vi "LabVIEW_commandline.vi"() -> ()   [LabVIEW 2016]
panel:
  out "concatenated string":string
  in  "Computer Selector":u16(ring)=1 items=["AERO-06", "AERO-03"]
  in  "PD Filepath":path=path "D:/PDE Project/PDE Data/Default Data/PD.tdms"
  in  "TC Filepath":path=path "D:/PDE Project/PDE Data/Default Data/TC.tdms"
  in  "PT Filepath":path=path "D:/PDE Project/PDE Data/Default Data/PT.tdms"
  in  "Diluent":string="N2"
  in  "Menu Ring":u16(ring) items=["Manual Find", "Use Path"]
  in  "Working Directory":path=path "C:/Users/DAQ/Desktop/Mass-Flow-Calculator"
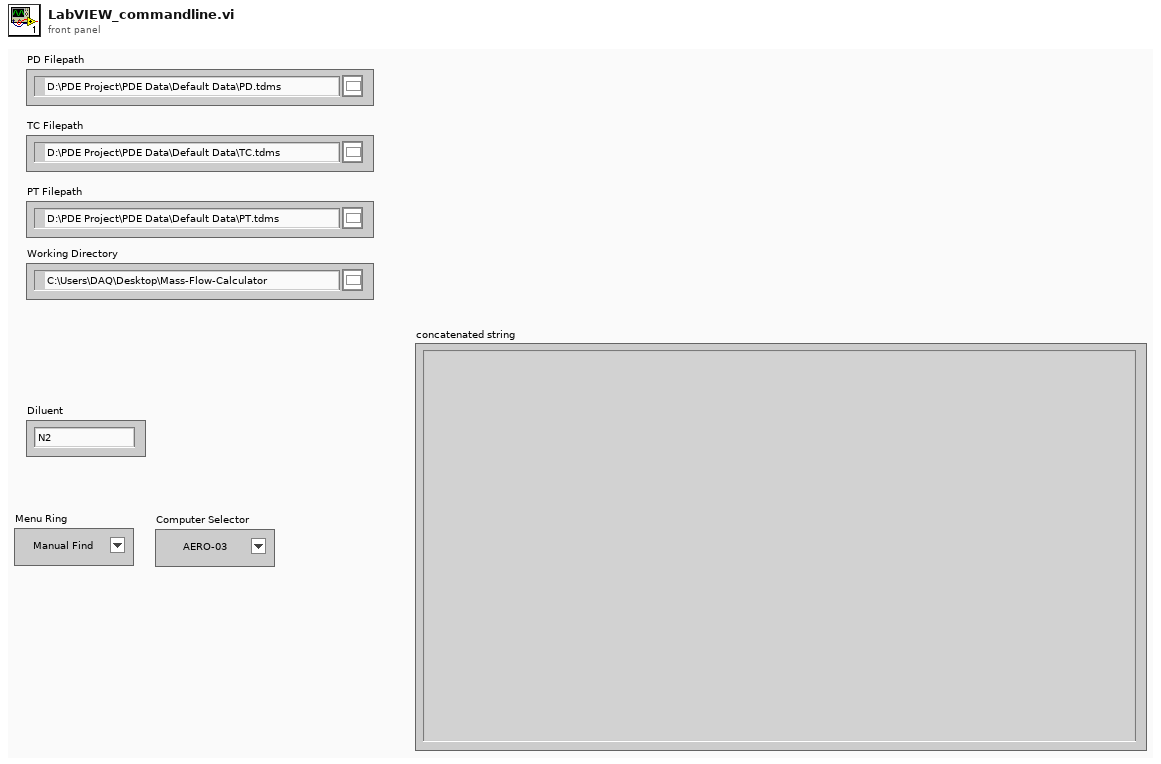
[diagram p1: front panel]
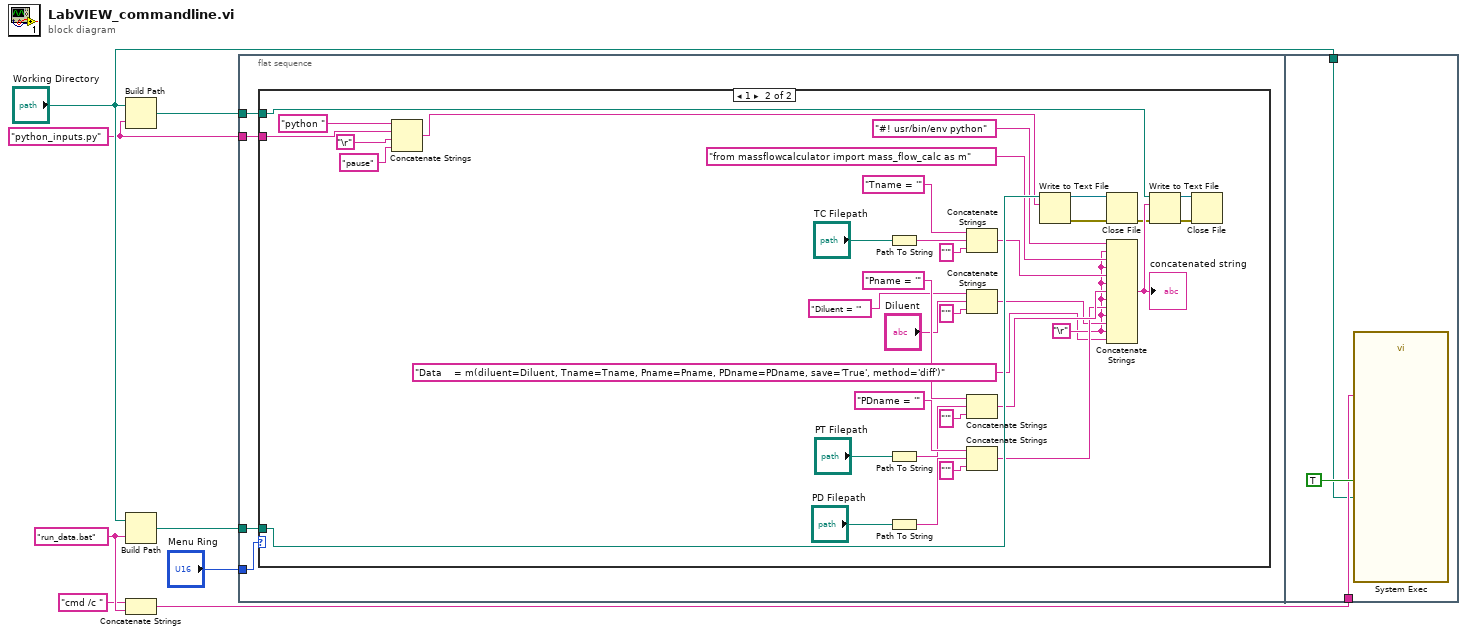
[diagram p0: block diagram]
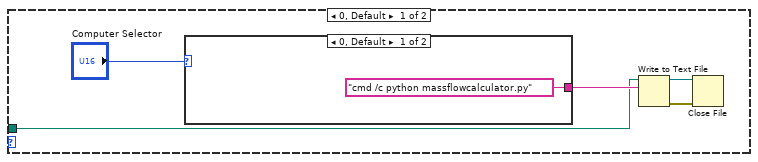
[diagram p2: hidden frame]
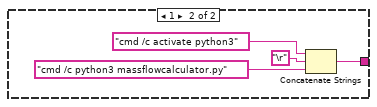
[diagram p3: hidden frame]
diagram:
  w1 = "python_inputs.py" ("name or relative path")
  w5 = "run_data.bat"
  n1 = Build Path(base path="Working Directory", name or relative path=w1) -> (appended path=w2:path)
  n2 = Build Path(base path="Working Directory", name or relative path=w5) -> (appended path=w7:path)
  n3 = Concatenate Strings("cmd /c " ("string"), w5) -> (w6:string)
  n4 = flat-sequence {
    tunnel: "Menu Ring" -> [w12]
    tunnel: w7 -> [w11]
    tunnel: w2 -> [w10]
    tunnel: w1 -> [w9]
    tunnel: w6 -> [w60]
    tunnel: "Working Directory" -> [w59]
    frame #0 {
      n5 = case shown="1" w12 {
        tunnel: w11 -> [w14 w53]
        tunnel: w10 -> [_ w28]
        tunnel: w9 -> [_ w26]
        frame 0, Default {
          n6 = case shown="0, Default" "Computer Selector" {
            tunnel: ["cmd /c python massflowcalculator.py" w19] -> w15
            frame 0, Default {
            }
            frame 1 {
              n7 = Concatenate Strings("cmd /c activate python3" ("text"), "\r", "cmd /c python3 massflowcalculator.py") -> (w19:string)
            }
          }
          n8 = Write to Text File(file (use dialog)=w14, text=w15) -> (refnum out=w16:refnum<file>, error out=w17:errorcluster)  [unwired: 2 in, 1 out]
          n9 = Close File(refnum=w16, error in=w17) -> ()  [unwired: 2 out]
        }
        frame 1 {
          w32 = "\r"
          n10 = Concatenate Strings("python " ("text"), w26, "\r", "pause" ("string")) -> (w25:string)
          n11 = Path To String(path="TC Filepath") -> (string=w46:string)
          n12 = Path To String(path="PT Filepath") -> (string=w41:string)
          n13 = Path To String(path="PD Filepath") -> (string=w40:string)
          n14 = Concatenate Strings("Tname = '" ("string"), w46, "'" ("string")) -> (w39:string)
          n15 = Concatenate Strings("Diluent = '" ("string"), "Diluent", "'" ("string")) -> (w33:string)
          n16 = Concatenate Strings("Pname = '" ("string"), w41, "'" ("string")) -> (w38:string)
          n17 = Concatenate Strings("PDname = '" ("string"), w40, "'" ("string")) -> (w37:string)
          n18 = Write to Text File(file (use dialog)=w53, text=w25) -> (refnum out=w54:refnum<file>, error out=w55:errorcluster)  [unwired: 2 in, 1 out]
          n19 = Close File(refnum=w54, error in=w55) -> (error out=w29:errorcluster)  [unwired: 1 out]
          n20 = Concatenate Strings("#! usr/bin/env python" ("string"), w32, "from massflowcalculator import mass_flow_calc as m" ("string"), w32, w39, w32, w38, w32, w37, w32, w33, w32, "Data    = m(diluent=Diluent, Tname=Tname, Pname=Pname, PDname=PDname, save='True', method='diff')" ("string")) -> (w30:string)
          "concatenated string" <- w30
          n21 = Write to Text File(file (use dialog)=w28, text=w30, error in=w29) -> (refnum out=w51:refnum<file>, error out=w52:errorcluster)  [unwired: 1 in, 1 out]
          n22 = Close File(refnum=w51, error in=w52) -> ()  [unwired: 2 out]
        }
      }
    }
    frame #1 {
      n23 = call <vilib>:"System Exec.vi"("wait until completion? (T)"=TRUE, "working directory"=w59, "command line"=w60) -> ()  [unwired: 5 in, 4 out]
    }
  }
